vi "Replace Custom Device VIs (SubVI).vi"(8 "error out":errorcluster, 10 "Custom Device Name":string, 11 "Custom Device Folder":path) -> (0 "error out 2":errorcluster, 3 "Custom Device VIs":path[](array[path]))   [LabVIEW 2010]
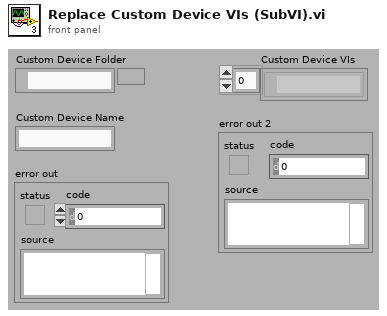
[diagram p1: front panel]
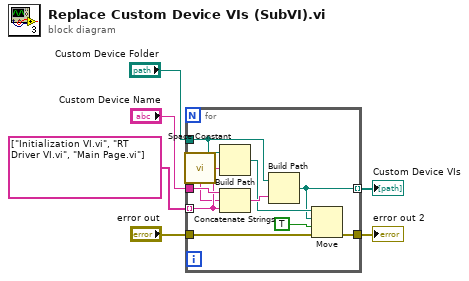
[diagram p0: block diagram]
diagram:
  n1 = for {
    tunnel: "Custom Device Folder" -> [w12]
    tunnel: "Custom Device Name" -> [w15]
    tunnel: string[] ["Initialization VI.vi", "RT Driver VI.vi", "Main Page.vi"] -> [w8] mode=indexing
    tunnel: "error out" -> [w14]
    tunnel: [w11] -> w2
    tunnel: [w9] -> w4 mode=indexing
    n2 = call <vilib>:"Space Constant.vi"() -> ("String"=w7:string)
    n3 = Build Path(base path=w12, name or relative path=w8) -> (appended path=w10:path)
    n4 = Concatenate Strings(w15, w7, w8) -> (w16:string)
    n5 = Build Path(base path=w12, name or relative path=w16) -> (appended path=w9:path)
    n6 = Move(source path=w10, error in=w14, 9:TRUE ("overwrite (F)"), 10:w9) -> (error out=w11:errorcluster)  [unwired: 1 in, 2 out]
  }
  "Custom Device VIs" <- w4
  "error out 2" <- w2
